vi "adjustdac.vi"(7 "input":dbl, 8 "down step":dbl, 9 "increase":bool, 10 "up step":dbl, 11 "decrease":bool) -> (2 "output":dbl)   [LabVIEW 2012]
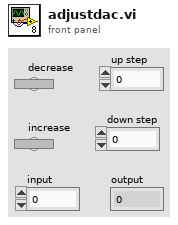
[diagram p1: front panel]
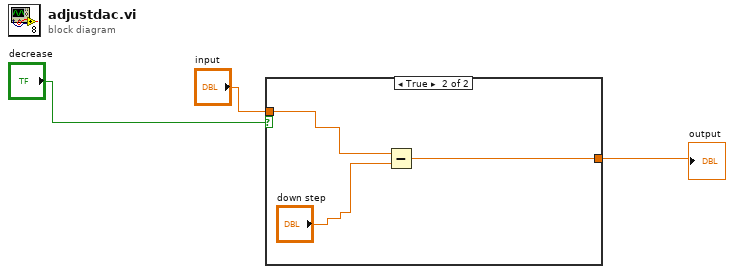
[diagram p0: block diagram]
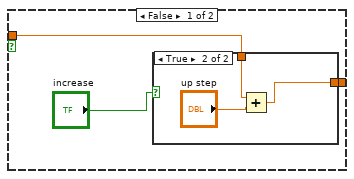
[diagram p2: hidden frame]
diagram:
  n1 = case shown="True" "decrease" {
    tunnel: "input" -> [w5 w13]
    tunnel: [w4 w12] -> w1
    frame False {
      n2 = case shown="True" "increase" {
        tunnel: w5 -> [w7 w9]
        tunnel: [w7 w10] -> w4
        frame False {
        }
        frame True {
          n3 = Add(x=w9, y="up step") -> (x+y=w10:dbl)
        }
      }
    }
    frame True {
      n4 = Subtract(x=w13, y="down step") -> (x-y=w12:dbl)
    }
  }
  "output" <- w1
